vi "Global_Bin_In_Var.vi"() -> ()   [LabVIEW 2016, in "DNP3_Master_Station_MGCC.lvlib"]
uses:
  <vilib>/DNP3/DNP3_Master/Poll Binary Input Variation.ctl
  DNP3_Master_Station_MGCC.lvlib
  <vilib>/DNP3/DNP3_Master.lvlib
panel:
  in  "Binary In Variation":T1 items=["Default", "Packed Format", "With Flags"]
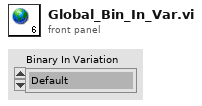
[diagram p1: front panel]
types:
  T1 = typedef "DNP3_Master.lvlib/Poll Binary Input Variation.ctl" = u8
diagram:
